vi "Tell.vi"(10 "Msg":refnum<class "Msg.lvclass">, 11 "Notifier Transport in":refnum<class "Notifier Transport.lvclass">) -> (0 "Error out":errorcluster)   [LabVIEW 2025, in "jettl.lvlib" / "Transport.lvlib" / "Notifier.lvlib" / "Notifier Transport.lvclass"]
uses:
  Notifier Transport.lvclass
  Msg/Msg.lvclass
  Notifier Transport.lvclass/Notifier Transport.ctl
  Teller/Teller.lvclass
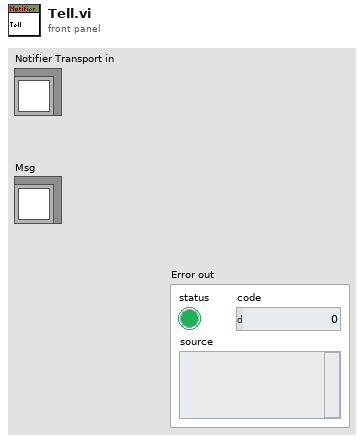
[diagram p1: front panel]
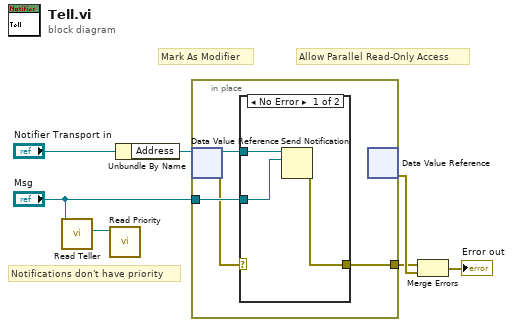
[diagram p0: block diagram]
diagram:
  # "Notifications don't have priority"
  # "Allow Parallel Read-Only Access"
  # "Mark As Modifier"
  n1 = call-dynamic "Read Teller.vi"("Msg in"="Msg") -> ("Teller"=w2:refnum<class "Teller.lvclass">)  [unwired: 10 in]
  n2 = call-dynamic "Read Priority.vi"("Teller in"=w2) -> ()  [unwired: 10 in, 1 out]
  n3 = Unbundle By Name("Notifier Transport in") -> ("Address"=w7:refnum<data-value>)
  n4 = in-place {
    in-place-border: [w11] -> w5
    in-place-border: "Msg" -> [w10]
    n5 = in-place-dvr #1(w7) -> (w9:refnum<notifier>, w8:errorcluster)
    n6 = case shown="No Error" w8 {
      selector: w8 -> [_ w15]
      tunnel: [w12 w15] -> w11
      tunnel: w10 -> [w13 _]
      tunnel: w9 -> [w14 _]
      frame No Error {
        n7 = Send Notification(notification=w13, notifier=w14) -> (error out=w12:errorcluster)  [unwired: 1 in, 1 out]
      }
      frame Error {
      }
    }
    n8 = in-place-dvr #1() -> (w6:errorcluster)  [unwired: 1 in, 1 out]
  }
  n9 = Merge Errors(w5, w6) -> (→"Error out":errorcluster)
